vi "(SubVI) Slowly Go to Target Posiiton_YCC.vi"(4 "scan rate  (um/s)":dbl=2.0 format="%.3f", 5 "axis":u32=1, 6 "Target position (um)":dbl) -> (0 "Expect - Real move (nm)\nStage Offset\n+=more move\n-=less move":dbl, 1 "step size (nm)":dbl, 2 "Now position (um)":dbl, 3 "True rate?":bool)   [LabVIEW 2014]
panel:
  out "traveling time (s)":dbl
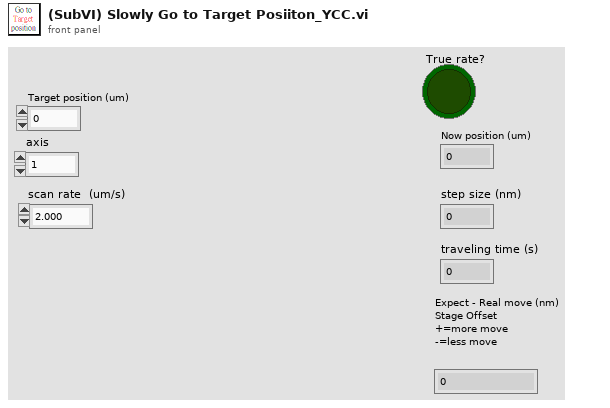
[diagram p1: front panel]
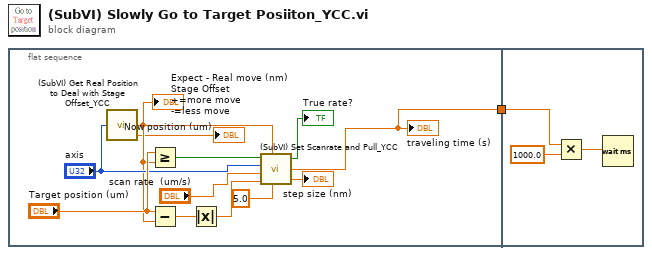
[diagram p0: block diagram]
diagram:
  n1 = flat-sequence {
    tunnel: [w3] -> w1
    tunnel: w1 -> [w14]
    frame #0 {
      n2 = call "(SubVI) Get Real Position to Deal with Stage Offset_YCC.vi"("Axis"="axis") -> ("Expect - Real move (nm)\nStage Offset\n+=more move\n-=less move"=→"Expect - Real move (nm)\nStage Offset\n+=more move\n-=less move":dbl, "Real Current Commanded position (um)"=w5:dbl)  [unwired: 3 in]
      "Now position (um)" <- w5
      n3 = Greater Or Equal?(x="Target position (um)", y=w5) -> (x >= y?=w13:bool)
      n4 = Subtract(x="Target position (um)", y=w5) -> (x-y=w11:dbl)
      n5 = Absolute Value(x=w11) -> (abs(x)=w10:dbl)
      n6 = call "(SubVI) Set Scanrate and Pull_YCC.vi"("toward+ ?\nT=+, F=-"=w13, "Start From  (um)"=w5, "axis"="axis", "scan rate  (um/s)"="scan rate  (um/s)", "waiting time per point (ms)\nrange from 5ms to 0.167 ms"=5.0 ("waiting time per point (ms)\nrange from 5ms to 0.167 ms"), "range  (um)"=w10) -> ("True rate?"=→"True rate?":bool, "traveling time (s)"=w3:dbl, "step size (nm)"=→"step size (nm)":dbl)
      "traveling time (s)" <- w3
    }
    frame #1 {
      n7 = Multiply(x=w14, y=1000.0) -> (x*y=w16:dbl)
      n8 = Wait (ms)(milliseconds to wait=w16) -> ()  [unwired: 1 out]
    }
  }
